vi "Define Table Row from Click Position.vi"(8 "error in":errorcluster, 10 "Coords":T1, 11 "Table Ref":refnum<vi>) -> (0 "error out":errorcluster, 2 "Packet in Bytes":u8[](array[numeric]), 3 "Packet in String":string)   [LabVIEW 2025, in "Automotive Ethernet Bus Monitor UI.lvlib"]
doc: "Helps to define the current row from a mouse click coord."
uses:
  Automotive Ethernet Bus Monitor UI.lvlib
  <vilib>/Utility/miscctls.llb/LVPoint32TypeDef.ctl
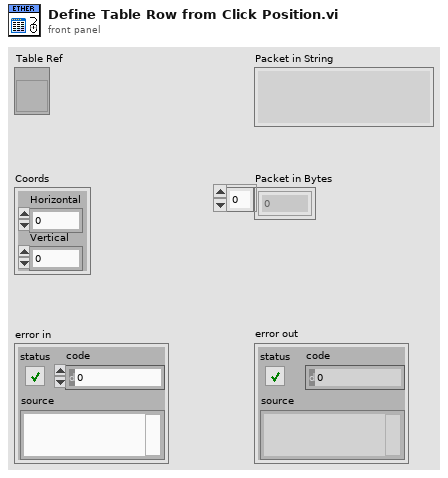
[diagram p1: front panel]
types:
  T1 = typedef "LVPoint32TypeDef.ctl" = cluster{"Horizontal":i32, "Vertical":i32}
  T2 = typedef "LVRowAndColumnTypeDef.ctl" = cluster{"Row":i32, "Column":i32}
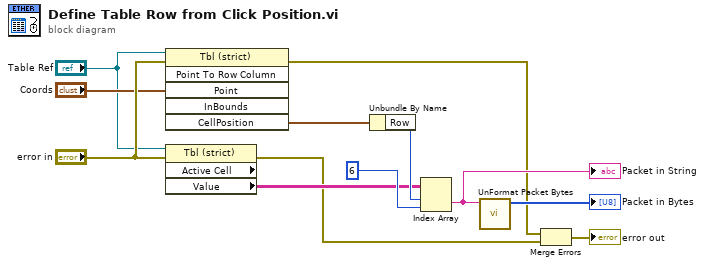
[diagram p0: block diagram]
diagram:
  n1 = invoke on="Invoke Node" class="Tbl (strict)" method="Point To Row Column"(reference="Table Ref", error in="error in", "Point"="Coords") -> (error out=w2:errorcluster, "CellPosition"=w9:T2)  [unwired: 3 in, 4 out]
  n2 = property on="Property Node" class="Tbl (strict)" props=["Active Cell", "Value"](reference="Table Ref", error in="error in") -> (error out=w3:errorcluster, "Value"=w5:string[][])  [unwired: 2 out]
  n3 = Unbundle By Name(w9) -> ("Row"=w7:i32)
  n4 = Index Array(array=w5, index (row)=w7, index (col)=6 ("disabled index (col)")) -> (element=w12:string)
  "Packet in String" <- w12
  n5 = call "UnFormat Packet Bytes.vi"("spreadsheet string"=w12) -> ("array"=→"Packet in Bytes":u8[])  [unwired: 10 in]
  n6 = Merge Errors(w2, w3) -> (→"error out":errorcluster)
